vi "classes.vi"(0 "HGF_Factory":refnum<class "HGF_Factory.lvclass">, 1 "className":string, 5 "error in (no error)":errorcluster) -> (14 "HGF_Factory dup":refnum<class "HGF_Factory.lvclass">, 16 "Object":refnum<class>, 19 "error out":errorcluster)   [LabVIEW 2014, in "HGF_BaseClasses.lvlib" / "HGF_Factory.lvclass"]
doc: "This dynamaic dispatch VI contains constant objects of all classes that can be produced by HGF_Factory.\nClass has to be defined by name. \n\nOptionally, you can also specifiy a Class Path String instead, but you have to make sure that all dependencies are available.\n\nChild classes have to override it to define additional classes."
uses:
  HGF_Factory.lvclass
  HGF_Base/HGF_Base.lvclass
  HGF_Composite/HGF_Composite.lvclass
  HGF_ThreadPool/HGF_ThreadPool.lvclass
  HGF_ThreadWorker/HGF_ThreadWorker.lvclass
  HGF_NextMultiple/HGF_NextMultiple.lvclass
  HGF_Wait/HGF_Wait.lvclass
  HGF_Queue/HGF_Queue.lvclass
  HGF_Occurrence/HGF_Occurrence.lvclass
  HGF_Notifier/HGF_Notifier.lvclass
  HGF_Rendezvous/HGF_Rendezvous.lvclass
  HGF_TaskOnce/HGF_TaskOnce.lvclass
  HGF_TaskLoop/HGF_TaskLoop.lvclass
  HGF_Stop/HGF_Stop.lvclass
  HGF_NetworkVisitor/HGF_NetworkVisitor.lvclass
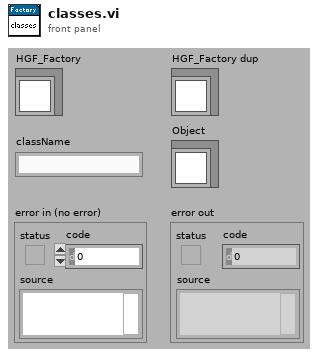
[diagram p1: front panel]
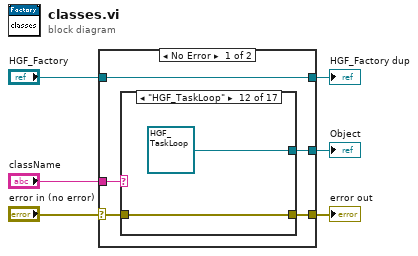
[diagram p0: block diagram]
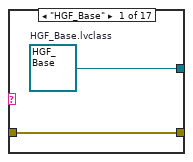
[diagram p2: hidden frame]
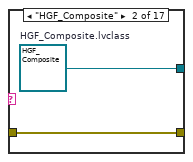
[diagram p3: hidden frame]
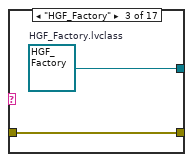
[diagram p4: hidden frame]
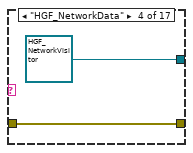
[diagram p5: hidden frame]
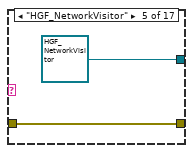
[diagram p6: hidden frame]
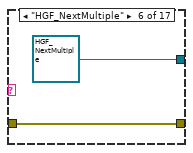
[diagram p7: hidden frame]
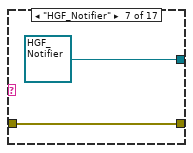
[diagram p8: hidden frame]
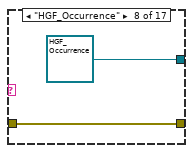
[diagram p9: hidden frame]
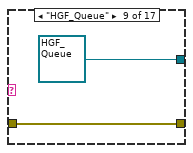
[diagram p10: hidden frame]
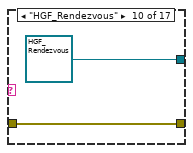
[diagram p11: hidden frame]
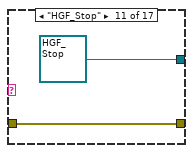
[diagram p12: hidden frame]
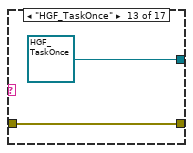
[diagram p13: hidden frame]
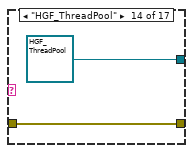
[diagram p14: hidden frame]
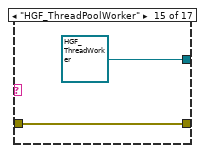
[diagram p15: hidden frame]
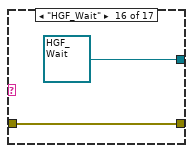
[diagram p16: hidden frame]
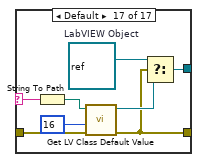
[diagram p17: hidden frame]
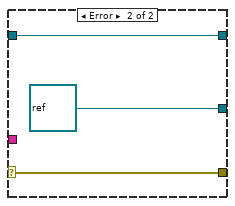
[diagram p18: hidden frame]
diagram:
  n1 = case shown="No Error" "error in (no error)" {
    selector: "error in (no error)" -> [w8 w54]
    tunnel: [w7 w54] -> w5
    tunnel: [w11 w53] -> w3
    tunnel: "HGF_Factory" -> [w11 w53]
    tunnel: "className" -> [w10 _]
    tunnel: [w9 refnum<class> refnum ("LabVIEW Object")] -> w1
    frame No Error {
      n2 = case shown="\"HGF_TaskLoop\"" w10 {
        selector: w10 -> [_ _ _ _ _ _ _ _ _ _ _ _ _ _ _ _ w49]
        tunnel: [w13 w15 w17 refnum<class "HGF_NetworkVisitor.lvclass"> refnum ("HGF_BaseClasses.lvlib:HGF_NetworkData.lvclass") refnum<class "HGF_NetworkVisitor.lvclass"> refnum ("HGF_BaseClasses.lvlib:HGF_NetworkVisitor.lvclass") refnum<class "HGF_NextMultiple.lvclass"> refnum ("HGF_BaseClasses.lvlib:HGF_NextMultiple.lvclass") refnum<class "HGF_Notifier.lvclass"> refnum ("HGF_BaseClasses.lvlib:HGF_Notifier.lvclass") refnum<class "HGF_Occurrence.lvclass"> refnum ("HGF_BaseClasses.lvlib:HGF_Occurrence.lvclass") refnum<class "HGF_Queue.lvclass"> refnum ("HGF_BaseClasses.lvlib:HGF_Queue.lvclass") refnum<class "HGF_Rendezvous.lvclass"> refnum ("HGF_BaseClasses.lvlib:HGF_Rendezvous.lvclass") refnum<class "HGF_Stop.lvclass"> refnum ("HGF_BaseClasses.lvlib:HGF_Stop.lvclass") refnum<class "HGF_TaskLoop.lvclass"> refnum ("HGF_BaseClasses.lvlib:HGF_ThreadTaskLoop.lvclass") refnum<class "HGF_TaskOnce.lvclass"> refnum ("HGF_BaseClasses.lvlib:HGF_ThreadTaskOnce.lvclass") refnum<class "HGF_ThreadPool.lvclass"> refnum ("HGF_BaseClasses.lvlib:HGF_ThreadPool.lvclass") refnum<class "HGF_ThreadWorker.lvclass"> refnum ("HGF_BaseClasses.lvlib:HGF_ThreadPoolWorker.lvclass") refnum<class "HGF_Wait.lvclass"> refnum ("HGF_BaseClasses.lvlib:HGF_Wait.lvclass") w50] -> w9
        tunnel: w8 -> [w12 w14 w16 w18 w20 w22 w24 w26 w28 w30 w32 w34 w36 w38 w40 w42 w44]
        tunnel: [w12 w14 w16 w18 w20 w22 w24 w26 w28 w30 w32 w34 w36 w38 w40 w42 w45] -> w7
        frame "HGF_Base" {
          w13 = refnum<class "HGF_Base.lvclass"> refnum  # HGF_Base.lvclass
        }
        frame "HGF_Composite" {
          w15 = refnum<class "HGF_Composite.lvclass"> refnum  # HGF_Composite.lvclass
        }
        frame "HGF_Factory" {
          w17 = refnum<class "HGF_Factory.lvclass"> refnum  # HGF_Factory.lvclass
        }
        frame "HGF_NetworkData" {
        }
        frame "HGF_NetworkVisitor" {
        }
        frame "HGF_NextMultiple" {
        }
        frame "HGF_Notifier" {
        }
        frame "HGF_Occurrence" {
        }
        frame "HGF_Queue" {
        }
        frame "HGF_Rendezvous" {
        }
        frame "HGF_Stop" {
        }
        frame "HGF_TaskLoop" {
        }
        frame "HGF_TaskOnce" {
        }
        frame "HGF_ThreadPool" {
        }
        frame "HGF_ThreadPoolWorker" {
        }
        frame "HGF_Wait" {
        }
        frame Default {
          w51 = refnum<class> refnum  # LabVIEW Object
          n3 = String To Path(string=w49) -> (path=w48:path)
          n4 = call <vilib>:"Get LV Class Default Value.vi"("error in (no error)"=w44, "options"=u32 16, "class path"=w48) -> ("error out"=w45:errorcluster, "object"=w46:refnum<class>)  [unwired: 7 out]
          n5 = Select(t=w51, s=w45, f=w46) -> (s? t:f=w50:refnum<class>)
        }
      }
    }
    frame Error {
    }
  }
  "error out" <- w5
  "HGF_Factory dup" <- w3
  "Object" <- w1
